vi "AcionaEletrovalvula.vi"(11 "queue Variaveis":refnum<queue>) -> ()   [LabVIEW 2018]
panel:
  in  "Stop":bool
  in  "Frequência":dbl
  in  "Duty Cycle %":dbl=50.0 min=0.0 max=100.0 step=1.0
  in  "Valvula in":bool=TRUE
  in  "Automático":bool
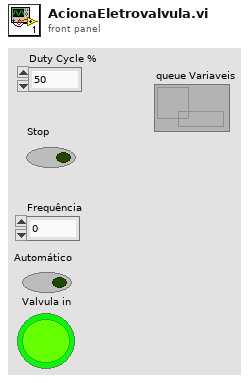
[diagram p1: front panel]
types:
  T1 = cluster{"Automatico":bool, "Valvula":bool, "Duty cycle":dbl, "Stop":bool, "Frequencia":dbl}
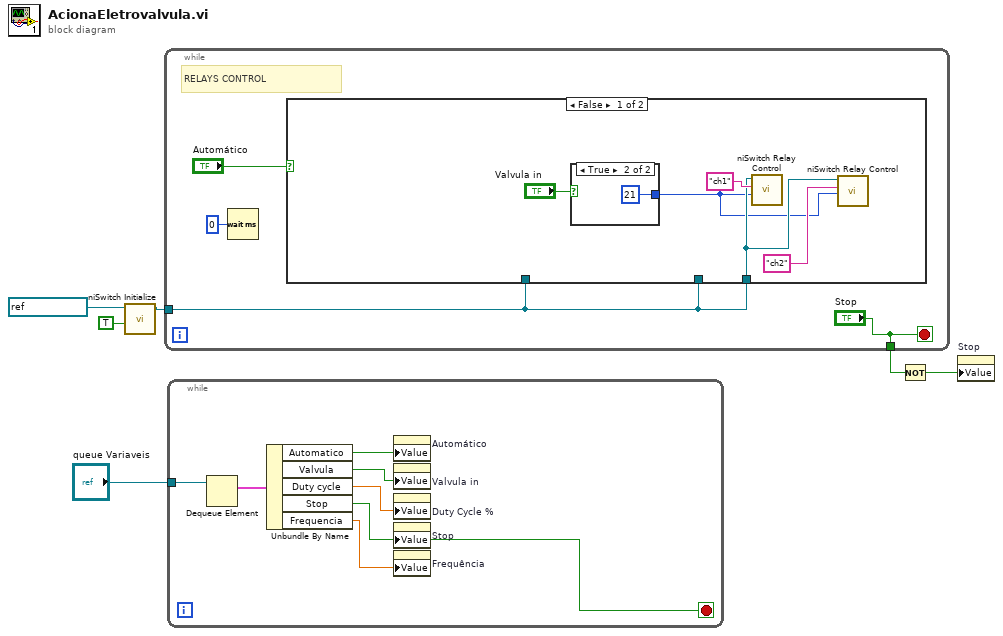
[diagram p0: block diagram]
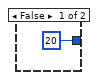
[diagram p2: hidden frame]
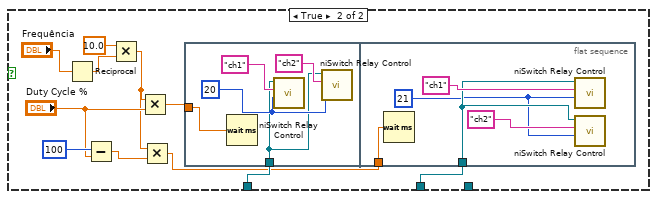
[diagram p3: hidden frame]
diagram:
  n1 = call <instrlib>:"niSwitch Initialize.vi"("reset device (boolean value)"=TRUE, "resource name"=refnum<k15> "SC1Mod3") -> ("instrument handle out"=w6:refnum<k15>)  [unwired: 8 in, 1 out]
  n2 = while {
    tunnel: w6 -> [w8]
    tunnel: ["Stop"] -> w3
    stop <- "Stop" stop-if-true
    # "RELAYS CONTROL"
    n3 = Wait (ms)(milliseconds to wait=u32 0) -> ()  [unwired: 1 out]
    n4 = case shown="False" "Automático" {
      tunnel: w8 -> [w12 _]
      tunnel: w8 -> [_ w28]
      tunnel: w8 -> [_ w27]
      frame False {
        n5 = case shown="True" "Valvula in" {
          tunnel: [20 21] -> w11
          frame False {
          }
          frame True {
          }
        }
        n6 = call <instrlib>:"niSwitch Relay Control.vi"("relay action (Close Relay)"=w11, "relay names"="ch1" ("String"), "instrument handle"=w12) -> ()  [unwired: 7 in, 2 out]
        n7 = call <instrlib>:"niSwitch Relay Control.vi"("relay action (Close Relay)"=w11, "relay names"="ch2" ("String"), "instrument handle"=w12) -> ()  [unwired: 7 in, 2 out]
      }
      frame True {
        n8 = Reciprocal(x="Frequência") -> (1/x=w26:dbl)
        n9 = Subtract(x=100, y="Duty Cycle %") -> (x-y=w21:dbl)
        n10 = Multiply(x=10.0 ("y"), y=w26) -> (x*y=w20:dbl)
        n11 = Multiply(x=w20, y="Duty Cycle %") -> (x*y=w24:dbl)
        n12 = Multiply(x=w20, y=w21) -> (x*y=w19:dbl)
        n13 = flat-sequence {
          tunnel: w28 -> [w29]
          tunnel: w24 -> [w32]
          tunnel: w27 -> [w35]
          tunnel: w19 -> [w37]
          frame #0 {
            w30 = 20
            n14 = Wait (ms)(milliseconds to wait=w32) -> ()  [unwired: 1 out]
            n15 = call <instrlib>:"niSwitch Relay Control.vi"("relay action (Close Relay)"=w30, "relay names"="ch1" ("String"), "instrument handle"=w29) -> ()  [unwired: 7 in, 2 out]
            n16 = call <instrlib>:"niSwitch Relay Control.vi"("relay action (Close Relay)"=w30, "relay names"="ch2" ("String"), "instrument handle"=w29) -> ()  [unwired: 7 in, 2 out]
          }
          frame #1 {
            w34 = 21
            n17 = Wait (ms)(milliseconds to wait=w37) -> ()  [unwired: 1 out]
            n18 = call <instrlib>:"niSwitch Relay Control.vi"("relay action (Close Relay)"=w34, "relay names"="ch1" ("String"), "instrument handle"=w35) -> ()  [unwired: 7 in, 2 out]
            n19 = call <instrlib>:"niSwitch Relay Control.vi"("relay action (Close Relay)"=w34, "relay names"="ch2" ("String"), "instrument handle"=w35) -> ()  [unwired: 7 in, 2 out]
          }
        }
      }
    }
  }
  n20 = while {
    tunnel: "queue Variaveis" -> [w45]
    stop <- w39 stop-if-true
    n21 = Dequeue Element(queue=w45) -> (element=w44:T1)  [unwired: 2 in, 3 out]
    n22 = Unbundle By Name(w44) -> ("Automatico"=w43:bool, "Valvula"=w42:bool, "Duty cycle"=w41:dbl, "Stop"=w39:bool, "Frequencia"=w40:dbl)
    n23 = property on="Automático" class="Bool (strict)"("Value"=w43) -> ()  [unwired: 2 in, 2 out]
    n24 = property on="Valvula in" class="Bool (strict)"("Value"=w42) -> ()  [unwired: 2 in, 2 out]
    n25 = property on="Duty Cycle %" class="DigNum (strict)"("Value"=w41) -> ()  [unwired: 2 in, 2 out]
    n26 = property on="Stop" class="Bool (strict)"("Value"=w39) -> ()  [unwired: 2 in, 2 out]
    n27 = property on="Frequência" class="DigNum (strict)"("Value"=w40) -> ()  [unwired: 2 in, 2 out]
  }
  n28 = Not(x=w3) -> (.not. x?=w2:bool)
  n29 = property on="Stop" class="Bool (strict)"("Value"=w2) -> ()  [unwired: 2 in, 2 out]
